vi "UNITTEST-JSON-RPC.vi"(8 "error in (no error)":errorcluster) -> (0 "error out":errorcluster)   [LabVIEW 2019]
uses:
  JSON-RPC/JSON-RPC.lvlib
  <vilib>/numeric/Random Number (Range) DBL.vi
  TEST-JSON-RPC--Cluster.ctl
  <vilib>/addons/_JKI Toolkits/Caraya/classes/Test/Test.lvclass
  <vilib>/addons/_JKI Toolkits/Caraya/classes/Assert/Assert.lvclass
  <vilib>/addons/_JKI Toolkits/Caraya/classes/Assert/Assert Almost Equal_Float.vi
  <vilib>/Utility/Data Type/NI_Data Type.lvlib
  bf96b4c4-93ca-40be-a8e5-266ffe2400d4.vi
  ff417335-71c0-49df-94a8-90e24726aa1e.vi
  79a25d12-cf8a-42c5-9792-37e3669560b3.vi
  a1349b84-7c34-4a80-901a-8b0d226f3268.vi
  458b24b7-cd46-4d6d-8e06-511d23d77ce6.vi
  6509a942-7c4c-4a72-a68d-56b70af1c45a.vi
  f131fd42-7747-4c67-9152-fee543478773.vi
  dfd8ca7f-1fc6-432d-8d21-06d145a1d0bd.vi
  a8a33294-d49e-44eb-9db6-4b34825de56e.vi
  d171704a-6168-4738-b7e5-c99b886d22e0.vi
  4b0d1cd5-144b-49c0-930c-ce61f585a09b.vi
panel:
  in  "wait (ms)":u32=1000
  out "Element (Request)":dbl[](array[numeric])
  out "Flatten (Request)":dbl[][](array[numeric])
  out "Flatten (Response)":dbl[][](array[numeric])
  out "Element (Response)":dbl[](array[numeric])
  out "Array (Request)":dbl[][](array[numeric])
  out "Cluster (Request)":T1[](array[typedef])
  out "Array (Response)":dbl[][](array[numeric])
  out "Cluster (Response)":T1[](array[typedef])
  out "Params":string[](array[string])
  out "Names":string[](array[string])
  out "REQ.Method":string
  out "<JSON> Response(s)":string
  out "<JSON> Request(s)":string
  out "4. parse response":dbl format="%#_6p"
  out "3. create response":dbl format="%#_6p"
  out "2. parse request":dbl format="%#_6p"
  out "1. create request":dbl format="%#_6p"
  out "REQ.Params":string
  out "results":string
  in  "Numeric":i32=3
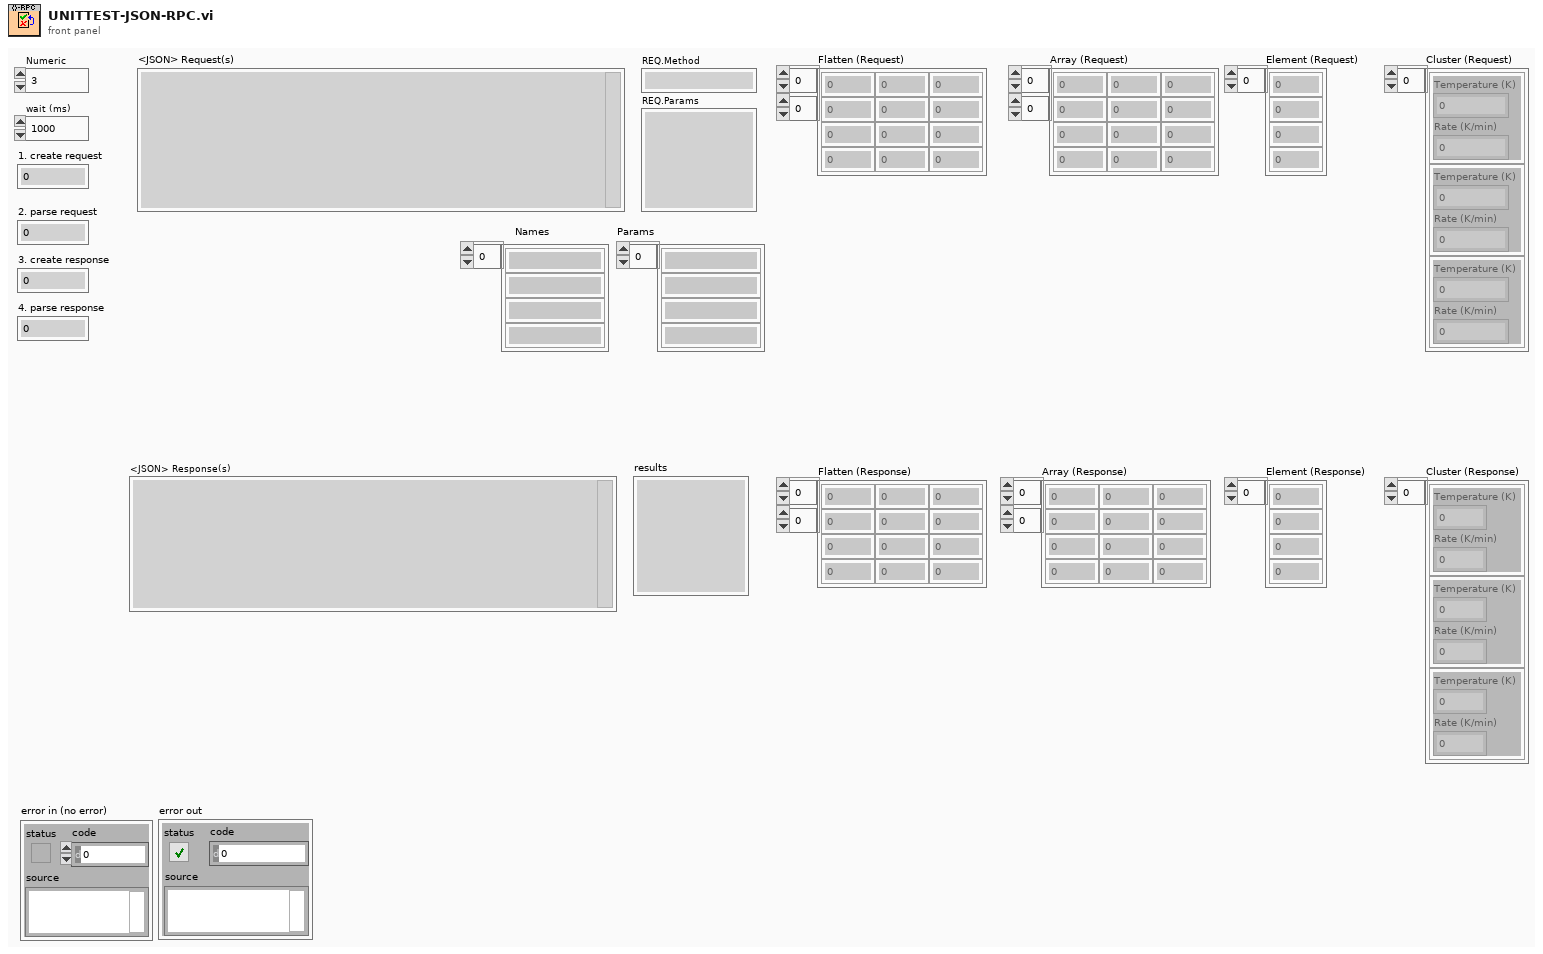
[diagram p1: front panel]
types:
  T1 = typedef "TEST-JSON-RPC--Cluster.ctl" = cluster{"Temperature (K)":dbl, "Rate (K/min)":dbl}
  T2 = enum16{"Parse Error", "Invalid Request", "Method not found", "Invalid params", "Internal error", "Server error"}
  T3 = cluster{"Temperature (K)":dbl, "Rate (K/min)":dbl}
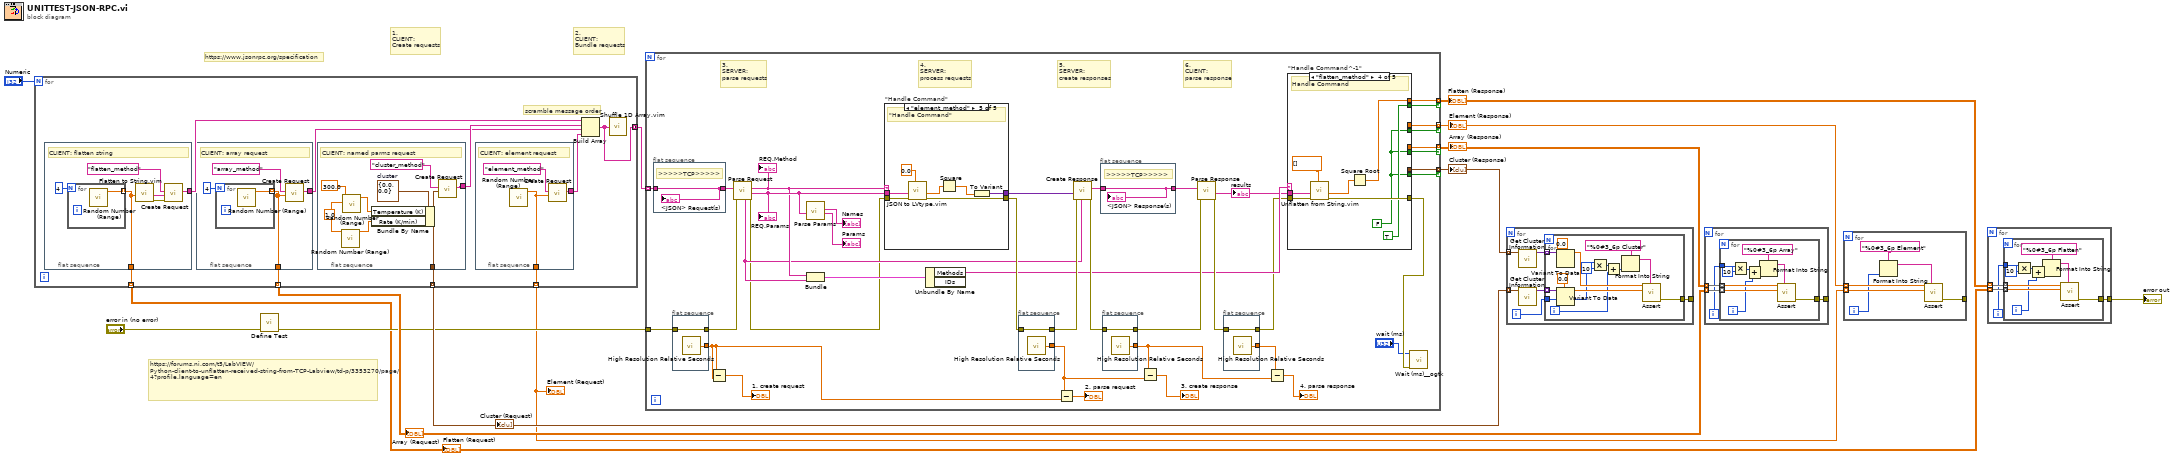
[diagram p0: block diagram]
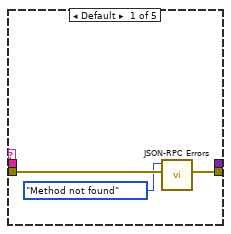
[diagram p2: hidden frame]
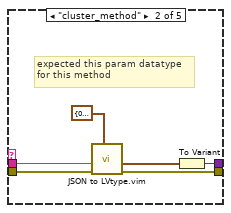
[diagram p3: hidden frame]
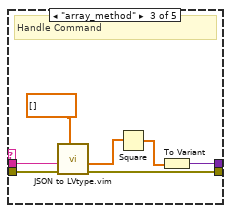
[diagram p4: hidden frame]
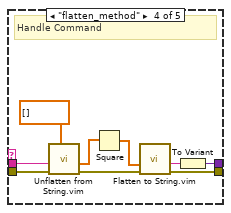
[diagram p5: hidden frame]
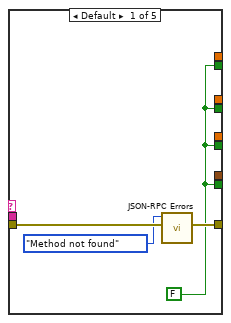
[diagram p6: hidden frame]
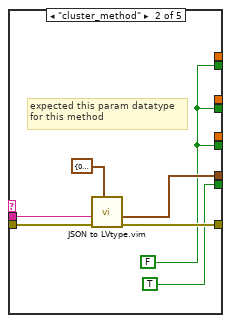
[diagram p7: hidden frame]
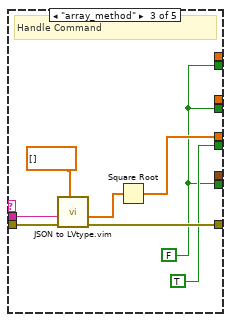
[diagram p8: hidden frame]
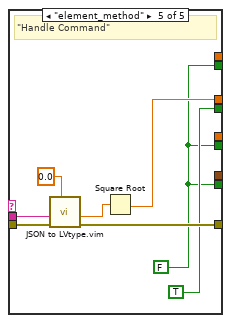
[diagram p9: hidden frame]
diagram:
  # "2.\nCLIENT:\nBundle requests"
  # "1.\nCLIENT:\nCreate requests"
  # "https://forums.ni.com/t5/LabVIEW/Python-client-to-unflatten-received-string-from-TCP-Labview/td-p/3353270/page/4?profile.language=en"
  # "https://www.jsonrpc.org/specification"
  n1 = for {
    N: "Numeric" -> [_]
    tunnel: [w14] -> w12 mode=concatenating
    tunnel: [w22] -> w10 mode=indexing
    tunnel: [w21] -> w9 mode=indexing
    tunnel: [w20] -> w1 mode=indexing
    tunnel: [w15] -> w2 mode=indexing
    # "scramble message order"
    n2 = flat-sequence {
      tunnel: [w27] -> w19
      tunnel: [w23] -> w15
      frame #0 {
        # "CLIENT: flatten string"
        n3 = for {
          N: 4 -> [_]
          tunnel: [w29] -> w23 mode=indexing
          n4 = call-poly <vilib>:"Random Number (Range).vi"() -> ("number"=w29:dbl)  [unwired: 11 in]
        }
        n5 = call "Flatten to String.vim"("Data in"=w23) -> ("error out"=w24:errorcluster, "<JSON>"=w25:string)  [unwired: 9 in]
        n6 = call "Create Request.vi"("error in (no error)"=w24, "params"=w25, "method"="flatten_method" ("Request.method")) -> ("<JSON> Requests"=w27:string)  [unwired: 5 in, 3 out]
      }
    }
    n7 = flat-sequence {
      tunnel: [w43] -> w17
      tunnel: [w41] -> w22
      frame #0 {
        # "CLIENT: array request"
        n8 = for {
          N: 4 -> [_]
          tunnel: [w45] -> w41 mode=indexing
          n9 = call-poly <vilib>:"Random Number (Range).vi"() -> ("number"=w45:dbl)  [unwired: 11 in]
        }
        n10 = call "Create Request.vi"("params"=w41, "method"="array_method" ("Request.method")) -> ("<JSON> Requests"=w43:string)  [unwired: 6 in, 3 out]
      }
    }
    n11 = flat-sequence {
      tunnel: [w37] -> w18
      tunnel: [w34] -> w21
      frame #0 {
        w38 = 1.0 ("lower bound (0)")
        w40 = T1 {"Temperature (K)"=0.0, "Rate (K/min)"=0.0}  # cluster
        # "CLIENT: named parms request"
        n12 = call-poly <vilib>:"Random Number (Range).vi"("upper bound (100)"=w38) -> ("number"=w36:dbl)  [unwired: 10 in]
        n13 = call-poly <vilib>:"Random Number (Range).vi"("lower bound (0)"=w38, "upper bound (100)"=300.0 ("lower bound (0)")) -> ("number"=w35:dbl)  [unwired: 9 in]
        n14 = Bundle By Name(cluster=w40, "Temperature (K)"=w35, "Rate (K/min)"=w36) -> (w34:T1)
        n15 = call "Create Request.vi"("params"=w34, "method"="cluster_method" ("Request.method")) -> ("<JSON> Requests"=w37:string)  [unwired: 6 in, 3 out]
      }
    }
    n16 = flat-sequence {
      tunnel: [w32] -> w16
      tunnel: [w31] -> w20
      frame #0 {
        # "CLIENT: element request"
        n17 = call-poly <vilib>:"Random Number (Range).vi"() -> ("number"=w31:dbl)  [unwired: 11 in]
        n18 = call "Create Request.vi"("params"=w31, "method"="element_method" ("Request.method")) -> ("<JSON> Requests"=w32:string)  [unwired: 6 in, 3 out]
      }
    }
    n19 = Build Array(w19, w18, w17, w16) -> (w14:string[])
    n20 = call "Shuffle 1D Array.vim"("array"=w14) -> ()  [unwired: 4 in, 1 out]
  }
  "Cluster (Request)" <- w9
  "Array (Request)" <- w10
  "Flatten (Request)" <- w2
  "Element (Request)" <- w1
  n21 = call <vilib>:"Define Test.vi"("error in (no error)"="error in (no error)") -> ("error out"=w7:errorcluster)  [unwired: 9 in, 1 out]
  n22 = for {
    tunnel: [w61] -> w8 mode=indexing if=w60
    tunnel: w12 -> [w72] mode=indexing
    tunnel: w7 -> [w50]
    tunnel: [w59] -> w5 mode=indexing if=w58
    tunnel: [w57] -> w4 mode=indexing if=w54
    tunnel: [w56] -> w6 mode=indexing if=w55
    # "3.\nSERVER:\nparse requests"
    # "6.\nCLIENT:\nparse response"
    # "4.\nSERVER:\nprocess requests"
    # "5.\nSERVER:\ncreate responses"
    n23 = flat-sequence {
      tunnel: w72 -> [w95]
      tunnel: [w95] -> w79
      frame #0 {
        # ">>>>>TCP>>>>>"
        "<JSON> Request(s)" <- w95
      }
    }
    n24 = flat-sequence {
      tunnel: [w92] -> w80
      tunnel: [w93] -> w51
      tunnel: w50 -> [w92]
      frame #0 {
        n25 = call <vilib>:"High Resolution Relative Seconds.vi"() -> ("relative seconds"=w93:dbl)
      }
    }
    n26 = Subtract(x=w51, y=w51) -> (x-y=→"1. create request":dbl)
    n27 = call "Parse Request.vi"("error in (no error)"=w80, "<JSON> Requests"=w79) -> ("error out"=w53:errorcluster, "Params"=w70:string, "Methods"=w67:string, "IDs"=w66:string)  [unwired: 5 in, 1 out]
    "REQ.Params" <- w70
    "REQ.Method" <- w67
    n28 = call "Parse Params.vi"("<JSON> Params"=w70) -> ("Params"=→"Params":string[], "Names"=→"Names":string[])  [unwired: 7 in, 2 out]
    n29 = Bundle("Methods"=w67, "IDs"=w66) -> (w65:cluster{"Methods":string, "IDs":string})  [unwired: 1 in]
    n30 = case "\"Handle Command\"" shown="\"element_method\"" w67 {
      tunnel: w53 -> [w98 w99 w110 w118 w123]
      tunnel: [w97 w100 w106 w113 w122] -> w84
      tunnel: [_ w104 w111 w120 w127] -> w71
      tunnel: w70 -> [_ w103 w109 w119 w125]
      frame Default {
        n31 = call "JSON-RPC Errors.vi"("error in"=w98, "Enum"=T2."Method not found") -> ("error out"=w97:errorcluster)  [unwired: 9 in]
      }
      frame "cluster_method" {
        # "expected this param datatype\nfor this method"
        n32 = call "JSON to LVtype.vim"("type"=T3 {"Temperature (K)"=0.0, "Rate (K/min)"=0.0} ("Cluster"), "error in (no error)"=w99, "JSON Data in"=w103) -> ("error out"=w100:errorcluster, "Data out"=w101:T3)  [unwired: 7 in]
        n33 = To Variant(anything=w101) -> (Variant=w104:variant)
      }
      frame "array_method" {
        # "Handle Command"
        n34 = call "JSON to LVtype.vim"("type"=dbl[] [] ("Numeric"), "error in (no error)"=w110, "JSON Data in"=w109) -> ("error out"=w106:errorcluster, "Data out"=w107:dbl[])  [unwired: 7 in]
        n35 = Square(x=w107) -> (x^2=w105:dbl[])
        n36 = To Variant(anything=w105) -> (Variant=w111:variant)
      }
      frame "flatten_method" {
        # "Handle Command"
        n37 = call "Unflatten from String.vim"("type"=dbl[] [] ("Numeric"), "error in (no error)"=w118, "<JSON>"=w119) -> ("error out"=w114:errorcluster, "Data out"=w117:dbl[])  [unwired: 7 in]
        n38 = Square(x=w117) -> (x^2=w115:dbl[])
        n39 = call "Flatten to String.vim"("error in (no error)"=w114, "Data in"=w115) -> ("error out"=w113:errorcluster, "<JSON>"=w112:string)  [unwired: 8 in]
        n40 = To Variant(anything=w112) -> (Variant=w120:variant)
      }
      frame "element_method" {
        # "\"Handle Command\""
        n41 = call "JSON to LVtype.vim"("type"=0.0 ("Numeric"), "error in (no error)"=w123, "JSON Data in"=w125) -> ("error out"=w122:errorcluster, "Data out"=w121:dbl)  [unwired: 7 in]
        n42 = Square(x=w121) -> (x^2=w126:dbl)
        n43 = To Variant(anything=w126) -> (Variant=w127:variant)
      }
    }
    n44 = Unbundle By Name(w65) -> ("Methods"=w64:string)  [unwired: 1 out]
    n45 = flat-sequence {
      tunnel: [w90] -> w74
      tunnel: [w91] -> w52
      tunnel: w84 -> [w90]
      frame #0 {
        n46 = call <vilib>:"High Resolution Relative Seconds.vi"() -> ("relative seconds"=w91:dbl)
      }
    }
    n47 = Subtract(x=w52, y=w51) -> (x-y=→"2. parse request":dbl)
    n48 = call "Create Response.vi"("id"=w66, "error in (no error)"=w74, "result"=w71) -> ("error out"=w73:errorcluster, "<JSON> Response"=w78:string)  [unwired: 6 in, 1 out]
    n49 = flat-sequence {
      tunnel: w78 -> [w94]
      tunnel: [w94] -> w75
      frame #0 {
        # ">>>>>TCP>>>>>"
        "<JSON> Response(s)" <- w94
      }
    }
    n50 = flat-sequence {
      tunnel: [w88] -> w77
      tunnel: [w89] -> w82
      tunnel: w73 -> [w88]
      frame #0 {
        n51 = call <vilib>:"High Resolution Relative Seconds.vi"() -> ("relative seconds"=w89:dbl)
      }
    }
    n52 = Subtract(x=w82, y=w52) -> (x-y=→"3. create response":dbl)
    n53 = call "Parse Response.vi"("error in (no error)"=w77, "<JSON> Response"=w75) -> ("error out"=w76:errorcluster, "results"=w62:string)  [unwired: 5 in, 3 out]
    "results" <- w62
    n54 = flat-sequence {
      tunnel: [w86] -> w63
      tunnel: [w87] -> w83
      tunnel: w76 -> [w86]
      frame #0 {
        n55 = call <vilib>:"High Resolution Relative Seconds.vi"() -> ("relative seconds"=w87:dbl)
      }
    }
    n56 = Subtract(x=w83, y=w82) -> (x-y=→"4. parse response":dbl)
    n57 = case "\"Handle Command^-1\"" shown="\"flatten_method\"" w64 {
      tunnel: w63 -> [w131 w135 w146 w153 w160]
      tunnel: [w130 w136 w142 w152 w159] -> w47
      tunnel: [_ w134 _ _ _] -> w61
      tunnel: w62 -> [_ w138 w145 w154 w162]
      tunnel: [w128 TRUE w139 w147 w155] -> w60
      tunnel: [_ _ w141 _ _] -> w59
      tunnel: [w128 w132 TRUE w147 w155] -> w58
      tunnel: [_ _ _ w149 _] -> w57
      tunnel: [_ _ _ _ w157] -> w56
      tunnel: [w128 w132 w139 w147 TRUE] -> w55
      tunnel: [w128 w132 w139 TRUE w155] -> w54
      frame Default {
        w128 = FALSE
        n58 = call "JSON-RPC Errors.vi"("error in"=w131, "Enum"=T2."Method not found") -> ("error out"=w130:errorcluster)  [unwired: 9 in]
      }
      frame "cluster_method" {
        w132 = FALSE
        # "expected this param datatype\nfor this method"
        n59 = call "JSON to LVtype.vim"("type"=T3 {"Temperature (K)"=0.0, "Rate (K/min)"=0.0} ("Cluster"), "error in (no error)"=w135, "JSON Data in"=w138) -> ("error out"=w136:errorcluster, "Data out"=w134:T3)  [unwired: 7 in]
      }
      frame "array_method" {
        w139 = FALSE
        # "Handle Command"
        n60 = call "JSON to LVtype.vim"("type"=dbl[] [] ("Numeric"), "error in (no error)"=w146, "JSON Data in"=w145) -> ("error out"=w142:errorcluster, "Data out"=w143:dbl[])  [unwired: 7 in]
        n61 = Square Root(x=w143) -> (sqrt(x)=w141:dbl[])
      }
      frame "flatten_method" {
        w147 = FALSE
        # "Handle Command"
        n62 = call "Unflatten from String.vim"("type"=dbl[] [] ("Numeric"), "error in (no error)"=w153, "<JSON>"=w154) -> ("error out"=w152:errorcluster, "Data out"=w151:dbl[])  [unwired: 7 in]
        n63 = Square Root(x=w151) -> (sqrt(x)=w149:dbl[])
      }
      frame "element_method" {
        w155 = FALSE
        # "\"Handle Command\""
        n64 = call "JSON to LVtype.vim"("type"=0.0 ("Numeric"), "error in (no error)"=w160, "JSON Data in"=w162) -> ("error out"=w159:errorcluster, "Data out"=w158:dbl)  [unwired: 7 in]
        n65 = Square Root(x=w158) -> (sqrt(x)=w157:dbl)
      }
    }
    n66 = call <userlib>:"Wait (ms)__ogtk.vi"("error in (no error)"=w47, "milliseconds to wait"="wait (ms)") -> ()  [unwired: 8 in, 2 out]
  }
  "Cluster (Response)" <- w8
  "Array (Response)" <- w5
  "Element (Response)" <- w6
  "Flatten (Response)" <- w4
  n67 = for {
    tunnel: w9 -> [w166] mode=indexing
    tunnel: [w168] -> _
    tunnel: w8 -> [w167] mode=indexing
    i -> [w163]
    n68 = call <vilib>:"Get Cluster Information.vi"("variant"=w167) -> ("cluster elements"=w164:variant[])  [unwired: 9 in, 1 out]
    n69 = call <vilib>:"Get Cluster Information.vi"("variant"=w166) -> ("cluster elements"=w165:variant[])  [unwired: 9 in, 1 out]
    n70 = for {
      tunnel: [w182] -> w168
      tunnel: w165 -> [w180] mode=indexing
      tunnel: w164 -> [w181] mode=indexing
      tunnel: w163 -> [w173]
      i -> [w172]
      n71 = Variant To Data(type=0.0, Variant=w181) -> (data=w176:dbl)  [unwired: 1 in, 1 out]
      n72 = Variant To Data(type=0.0, Variant=w180) -> (data=w179:dbl)  [unwired: 1 in, 1 out]
      n73 = Multiply(x=w173, y=10) -> (x*y=w175:i32)
      n74 = Add(x=w175, y=w172) -> (x+y=w171:i32)
      n75 = Format Into String(format string="%0#3_6p Cluster" ("Label"), w171) -> (resulting string=w170:string)  [unwired: 2 in, 1 out]
      n76 = call-poly <vilib>:"Assert.vi"("Label"=w170, "Y"=w179, "X"=w176) -> ("error out"=w182:errorcluster)  [unwired: 7 in, 1 out]
    }
  }
  n77 = for {
    tunnel: w10 -> [w186] mode=indexing
    tunnel: w5 -> [w185] mode=indexing
    tunnel: [w184] -> _
    i -> [w183]
    n78 = for {
      tunnel: w186 -> [w196] mode=indexing
      tunnel: w185 -> [w195] mode=indexing
      tunnel: [w194] -> w184
      tunnel: w183 -> [w191]
      i -> [w188]
      n79 = Multiply(x=w191, y=10) -> (x*y=w189:i32)
      n80 = Add(x=w189, y=w188) -> (x+y=w187:i32)
      n81 = Format Into String(format string="%0#3_6p Array" ("Label"), w187) -> (resulting string=w192:string)  [unwired: 2 in, 1 out]
      n82 = call-poly <vilib>:"Assert.vi"("Label"=w192, "Y"=w196, "X"=w195) -> ("error out"=w194:errorcluster)  [unwired: 7 in, 1 out]
    }
  }
  n83 = for {
    tunnel: w1 -> [w202] mode=indexing
    tunnel: w6 -> [w201] mode=indexing
    tunnel: [w200] -> _
    i -> [w199]
    n84 = Format Into String(format string="%0#3_6p Element" ("Label"), w199) -> (resulting string=w197:string)  [unwired: 2 in, 1 out]
    n85 = call-poly <vilib>:"Assert.vi"("Label"=w197, "Y"=w202, "X"=w201) -> ("error out"=w200:errorcluster)  [unwired: 7 in, 1 out]
  }
  n86 = for {
    tunnel: w2 -> [w206] mode=indexing
    tunnel: w4 -> [w205] mode=indexing
    tunnel: [w204] -> w3
    i -> [w203]
    n87 = for {
      tunnel: w206 -> [w216] mode=indexing
      tunnel: w205 -> [w215] mode=indexing
      tunnel: [w214] -> w204
      tunnel: w203 -> [w211]
      i -> [w208]
      n88 = Multiply(x=w211, y=10) -> (x*y=w209:i32)
      n89 = Add(x=w209, y=w208) -> (x+y=w207:i32)
      n90 = Format Into String(format string="%0#3_6p Flatten" ("Label"), w207) -> (resulting string=w212:string)  [unwired: 2 in, 1 out]
      n91 = call-poly <vilib>:"Assert.vi"("Label"=w212, "Y"=w216, "X"=w215) -> ("error out"=w214:errorcluster)  [unwired: 7 in, 1 out]
    }
  }
  "error out" <- w3
